vi "Close.vi"(8 "error in (no error)":errorcluster, 11 "CS++Method in":refnum<class "CS++Method.lvclass">) -> (0 "error out":errorcluster, 3 "CS++Method out":refnum<class "CS++Method.lvclass">)   [LabVIEW 2015, in "CS++Method.lvlib" / "CS++Method.lvclass"]
doc: "Removes the references to the Methods."
uses:
  CS++Method.lvclass
  CS++Method.lvclass/CS++Method.ctl
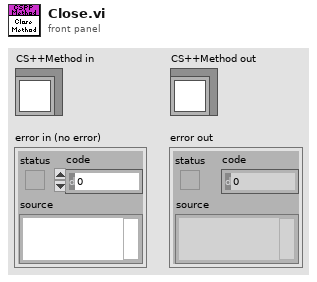
[diagram p1: front panel]
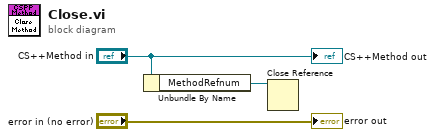
[diagram p0: block diagram]
diagram:
  n1 = Unbundle By Name("CS++Method in") -> ("MethodRefnum"=w1:refnum<vi>)
  n2 = Close Reference(reference=w1) -> ()  [unwired: 1 in, 1 out]
  "error out" <- "error in (no error)"
  "CS++Method out" <- "CS++Method in"
